vi "integra.vi"(8 "period":dbl, 11 "X":dbl) -> (3 "R":dbl)   [LabVIEW 2019]
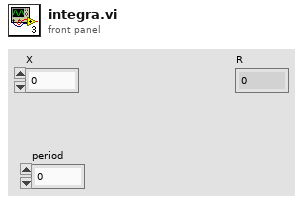
[diagram p1: front panel]
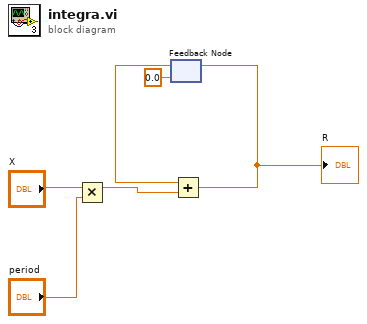
[diagram p0: block diagram]
diagram:
  n1 = Multiply(x="X", y="period") -> (x*y=w2:dbl)
  n2 = feedback #1(0.0) -> (w5:dbl)
  n3 = Add(x=w5, y=w2) -> (x+y=w3:dbl)
  "R" <- w3
  n4 = feedback-in #1(w3) -> ()
